vi "FilterMulti.vi"(9 "Error in":errorcluster, 10 "Codes to filter":i32[](array[numeric])) -> (1 "Error out":errorcluster, 2 "Code(s) filtered?":bool)   [LabVIEW 2017, in "GPError.lvlib"]
doc: "Clears the error or warning on <B>Error in</B> if Code in <B>Error in</B> matches any of the entries in <B>Codes to filter</B>.\n\nThis VI supports filtering appended errors, in which case it clears only those elements in the appended error collection that matches <B>Codes to filter</B>.\n\n<B>Code(s) filtered?</B> will be True only if <B>Error in</B> was filtered.\n\nThis VI is inlined.\n\nSteen Schmidt\nGPower\n18/7 2013"
uses:
  GPError.lvlib
panel:
  # "Copyright © 2013\nSteen Schmidt, GPower\nSee enclosed license file for terms and conditions"
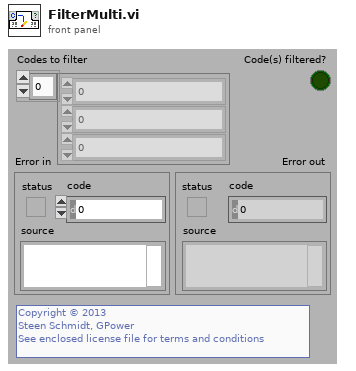
[diagram p1: front panel]
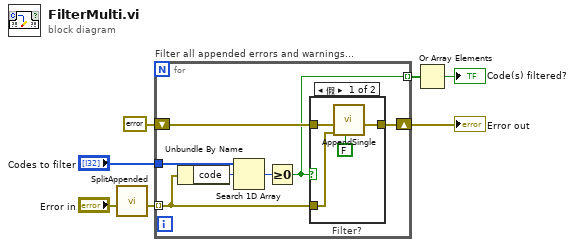
[diagram p0: block diagram]
diagram:
  n1 = call "SplitAppended.vi"("Appended errors in"="Error in") -> ("Errors out"=w7:errorcluster[])  [unwired: 10 in]
  n2 = for "Filter all appended errors and warnings..." {
    tunnel: w7 -> [w11] mode=indexing
    tunnel: "Codes to filter" -> [w13]
    shift-right: [w10] -> w3
    shift-left: errorcluster {"status"=FALSE, "code"=0, "source"=""} ("error out") -> [w12]
    tunnel: [w9] -> w5 mode=indexing
    n3 = Unbundle By Name(w11) -> ("code"=w14:i32)
    n4 = Search 1D Array(1D array=w13, element=w14) -> (index of element=w8:i32)  [unwired: 1 in]
    n5 = Greater Or Equal To 0?(x=w8) -> (x >= 0?=w9:bool)
    n6 = case "Filter?" shown="假" w9 {
      tunnel: w12 -> [w18 w19]
      tunnel: w11 -> [w17 _]
      tunnel: [w16 w19] -> w10
      frame False {
        n7 = call "AppendSingle.vi"("Only append if new?"=FALSE, "Error to append"=w17, "Error in"=w18) -> ("Appended errors out"=w16:errorcluster)  [unwired: 8 in]
      }
      frame True {
      }
    }
  }
  "Error out" <- w3
  n8 = Or Array Elements(Boolean array=w5) -> (logical OR=→"Code(s) filtered?":bool)
